vi "Pre Launch Init.vi"(11 "BoundViewManager in":refnum<class "BoundViewManager.lvclass">) -> (0 "error out":errorcluster, 3 "BoundViewManager out":refnum<class "BoundViewManager.lvclass">)   [LabVIEW 2017, in "BoundViewManager.lvlib" / "BoundViewManager.lvclass"]
doc: "(<B>Filename</B>: Actor Framework.lvlib:Actor.lvclass:Pre Launch Init.vi)\n\nDefines behavior that occurs after the Launch Nested Actor method is invoked but before the actor's Actor Core method begins running.\n\nBy default, this method does nothing. A descendant class may override it to define behavior.\n\n<License>\nCopyright © 2017 Composed Systems, LLC | All rights reserved\nwww.composed.io\n\nAuthor: Ethan Stern <ethan.stern@composed.io>\n\nThis software is provided \"AS IS\" WITHOUT WARRANTIES, either express or implied, AND IS FOR EDUCATIONAL PURPOSES ONLY.\n</License>"
uses:
  BoundViewManager.lvclass
  C:/Git/mva-framework/Framework/IObserver/IObserver/IObserver.lvclass
  BoundViewManager Messages/Insert Bound View Msg/Insert Bound View Msg.lvclass
  C:/Git/mva-framework/Framework/Transport/ActorMessageTransport/Notification Msg/Notification Msg.lvclass
  BoundViewManager.lvclass/BoundViewManager.ctl
  Framework/SubscriptionPolicy/BasicSubscription/BasicSubscription.lvclass/BasicSubscription.ctl
  Framework/SubscriptionPolicy/ValueChangeSubscription/ValueChangeSubscription.lvclass/ValueChangeSubscription.ctl
  Framework/SubscriptionPolicy/BasicSubscription/BasicSubscription.lvclass
  C:/Git/mva-framework/Framework/IMediator/ISubscriptionPolicy/ISubscriptionPolicy.lvclass
  Framework/SubscriptionPolicy/ValueChangeSubscription/ValueChangeSubscription.lvclass
  Framework/IViewManager/IViewManager/IViewManager.lvclass
  <vilib>/Composed Systems/Current Value Table/CurrentValueTable.lvclass
  Framework/IObserver/IObserver/IObserver.lvclass
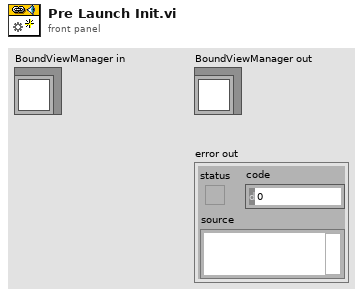
[diagram p1: front panel]
types:
  T1 = typedef "CurrentValueTable.lvlib/CurrentValueTable.lvclass/CurrentValueTable Reference.ctl" = refnum<data-value>
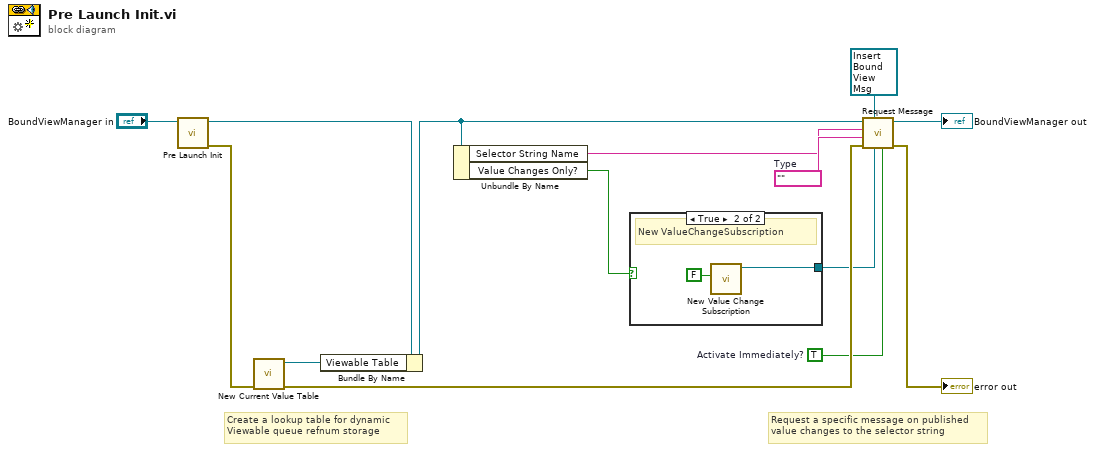
[diagram p0: block diagram]
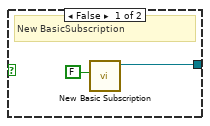
[diagram p2: hidden frame]
diagram:
  w3 = TRUE  # Activate Immediately?
  w6 = ""  # Type
  # "Request a specific message on published\nvalue changes to the selector string"
  # "Create a lookup table for dynamic\nViewable queue refnum storage"
  n1 = call-parent "Pre Launch Init.vi"("IViewManager in"="BoundViewManager in") -> ("error out"=w12:errorcluster, "IViewManager out"=w14:refnum<class "BoundViewManager.lvclass">)  [unwired: 9 in]
  n2 = call <vilib>:"New Current Value Table.vi"("error in (no error)"=w12) -> ("error out"=w9:errorcluster, "Current Value Table"=w11:T1)  [unwired: 9 in]
  n3 = Bundle By Name(cluster=w14, "Viewable Table"=w11) -> (w5:refnum<class "BoundViewManager.lvclass">)
  n4 = Unbundle By Name(w5) -> ("Selector String Name"=w4:string, "Value Changes Only?"=w2:bool)
  n5 = case shown="True" w2 {
    tunnel: [w16 w18] -> w1
    frame False {
      # "New BasicSubscription"
      n6 = call "New Basic Subscription.vi"("Ignore Past Updates? (F)"=FALSE) -> ("BasicSubscription Out"=w16:refnum<class "BasicSubscription.lvclass">)  [unwired: 10 in]
    }
    frame True {
      # "New ValueChangeSubscription"
      n7 = call "New Value Change Subscription.vi"("Ignore Past Updates? (F)"=FALSE) -> ("ValueChangeSubscription Out"=w18:refnum<class "ValueChangeSubscription.lvclass">)  [unwired: 10 in]
    }
  }
  n8 = call "Request Message.vi"("Activate Immediately? (T)"=w3, "SubscriptionPolicy"=w1, "Desired Notification Msg"=refnum<class "Insert Bound View Msg.lvclass"> refnum ("BoundViewManager.lvlib:Insert Bound View Msg.lvclass"), "error in (no error)"=w9, "Data Type"=w6, "Datum Name"=w4, "IObserver in"=w5) -> ("error out"=→"error out":errorcluster, "IObserver out"=→"BoundViewManager out":refnum<class "BoundViewManager.lvclass">)  [unwired: 2 in, 1 out]
